vi "Alphabet--constant.vi"() -> (2 "Alphabet (ASCII U8 values)":u8[](array[numeric]), 3 "Alphabet (lowercase strings)":string[](array[string])=["a", "b", "c", "d", "e", "f", "g", "h", "i", "j", "k", "l", "m", "n", "o", "p", "q", "r", "s", "t", "u", "v", "w", "x", "y", "z"])   [LabVIEW 2020, in "Wordle Engine.lvlib"]
doc: "Returns an array of characters representing the lowercase alphabet, from a to z. Also returns the U8 ASCII characters corresponding to each lowercase letter."
uses:
  Wordle Engine.lvlib
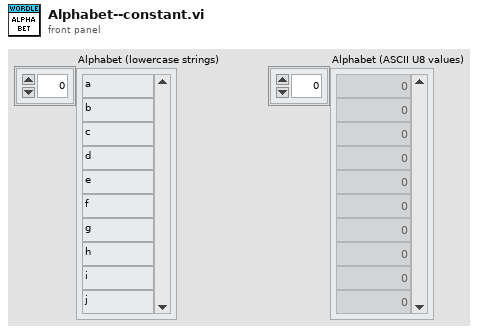
[diagram p1: front panel]
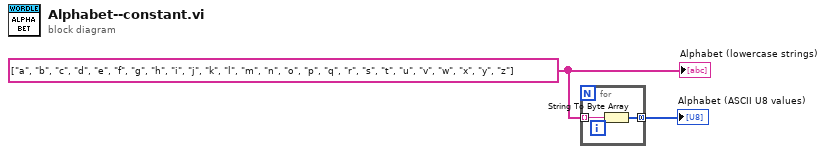
[diagram p0: block diagram]
diagram:
  w2 = string[] ["a", "b", "c", "d", "e", "f", "g", "h", "i", "j", "k", "l", "m", "n", "o", "p", "q", "r", "s", "t", "u", "v", "w", "x", "y", "z"]
  n1 = for {
    tunnel: w2 -> [w4] mode=indexing
    tunnel: [w3] -> w1 mode=concatenating
    n2 = String To Byte Array(string=w4) -> (unsigned byte array=w3:u8[])
  }
  "Alphabet (ASCII U8 values)" <- w1
  "Alphabet (lowercase strings)" <- w2
